vi "Read_Data_file.vi"(0 "Results file":path, 1 "Read Channel Names only":bool, 3 "Add Extra Channels?":bool, 5 "Template File":path, 8 "Desired File Types":T1) -> (10 "Row numbers":i32[](array[numeric]), 11 "Template File Out":path, 12 "Filetype":string, 13 "EOF?":bool, 14 "Results file Out":path, 15 "String Before":string, 16 "Ch names Out":string[](array[string]), 17 "Channel Values Out":string[][](array[string]), 18 "String After":string, 19 "mark after read (chars.)":i32)   [LabVIEW 2015]
uses:
  Data_File_Type.ctl
  Results_plotter_Global.vi
  Globals/Meas_global.vi
panel:
  out "Case":string
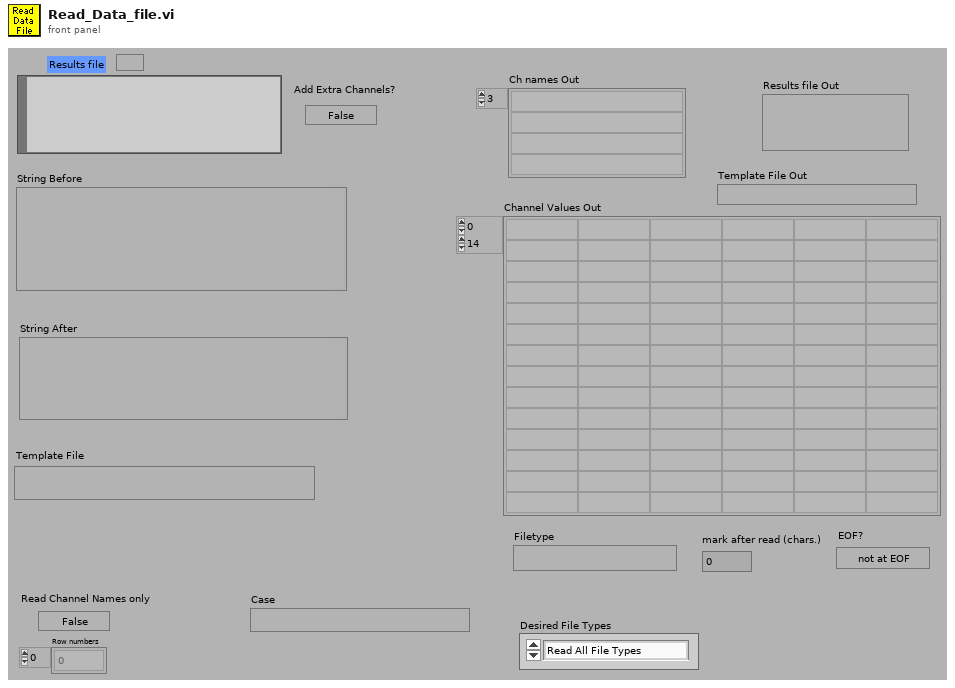
[diagram p1: front panel]
types:
  T1 = typedef "Data_File_Type.ctl" = enum16{"Read All File Types", "Results Files Only", "Raw Data Files Only", "Calibration Files Only", "Gas Desk Files Only", "Old Results Files Only", "Tabulated Data Files Only"}
  T2 = enum32{"existing file", "new file", "new or existing file", "existing dir", "new dir", "new or existing dir", "existing file (use LLBs)", "new file (use LLBs)", "new or existing file (use LLBs)", "new or existing file or directory (use LLBs)"}
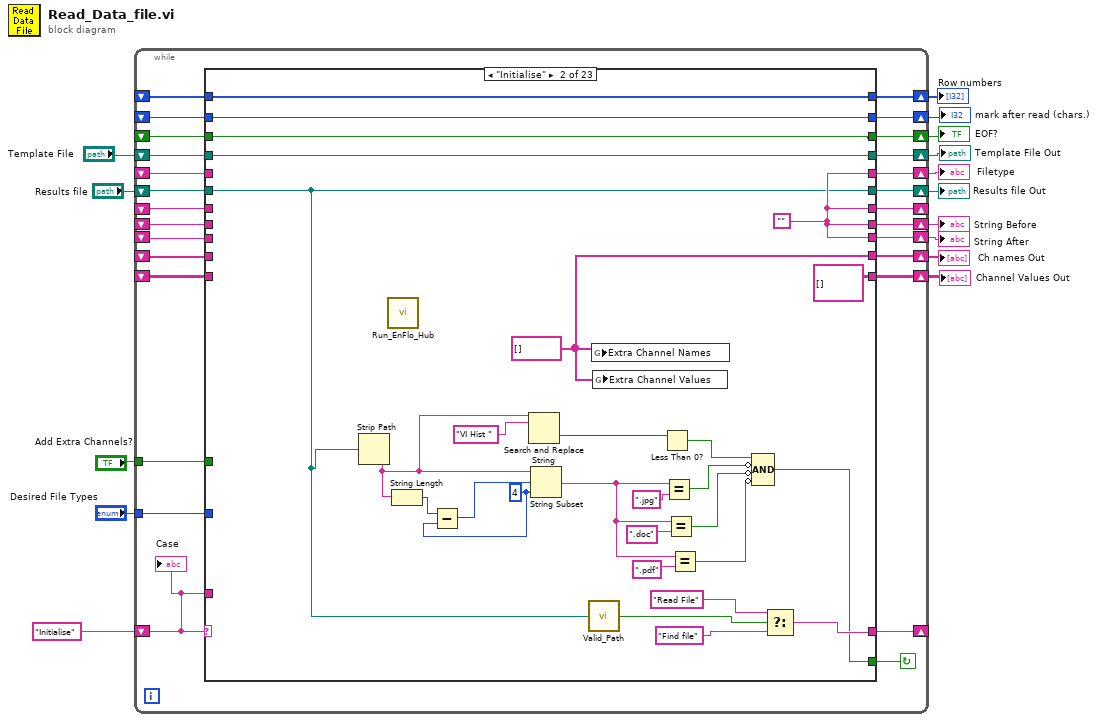
[diagram p0: block diagram]
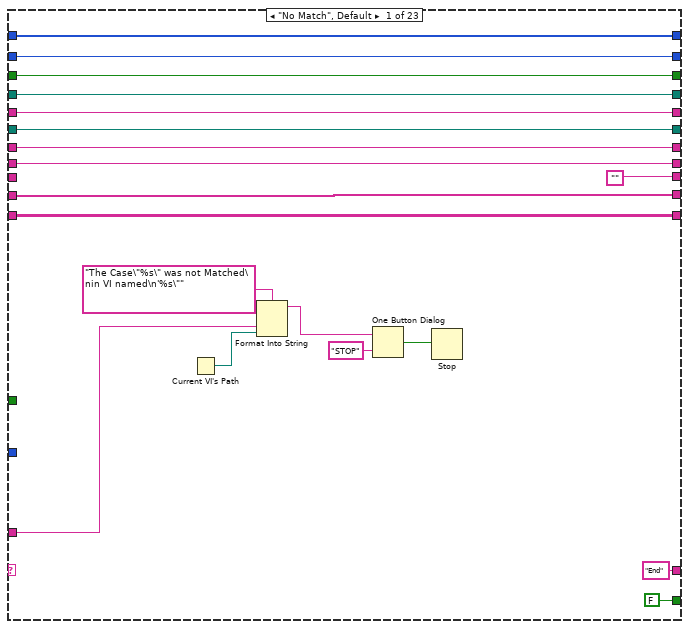
[diagram p2: hidden frame]
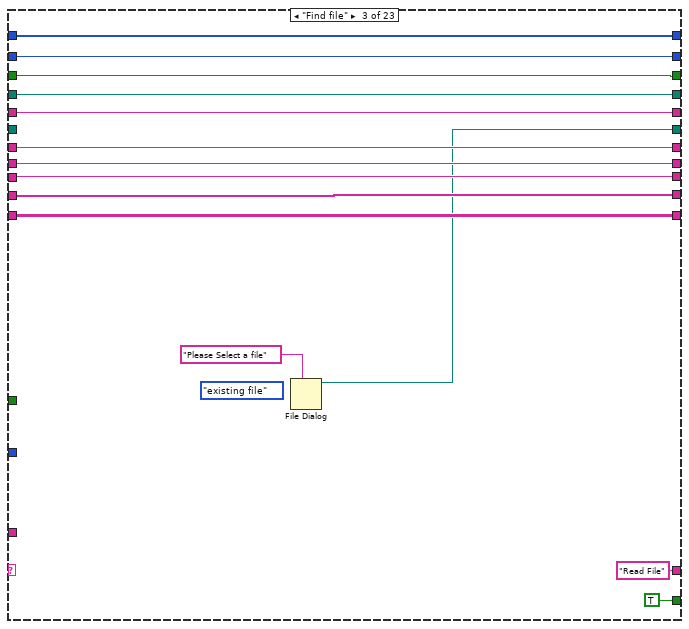
[diagram p3: hidden frame]
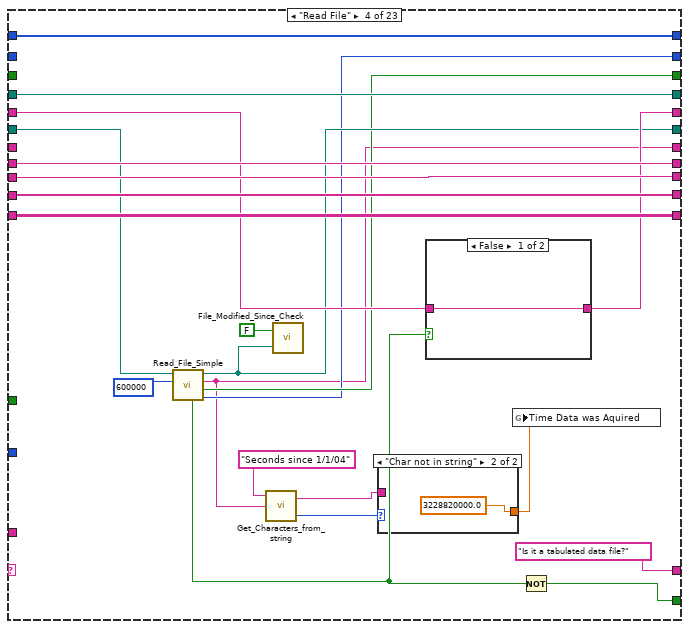
[diagram p4: hidden frame]
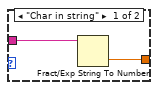
[diagram p5: hidden frame]
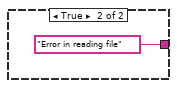
[diagram p6: hidden frame]
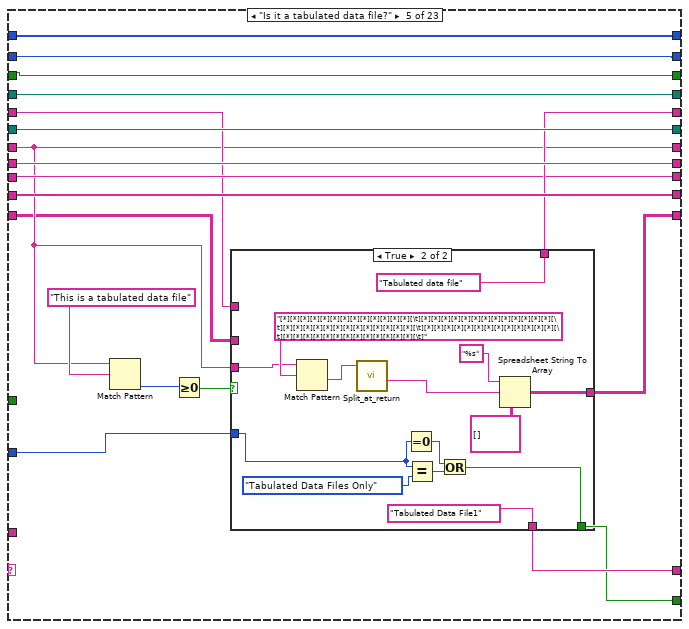
[diagram p7: hidden frame]
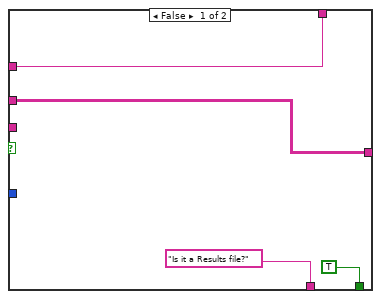
[diagram p8: hidden frame]
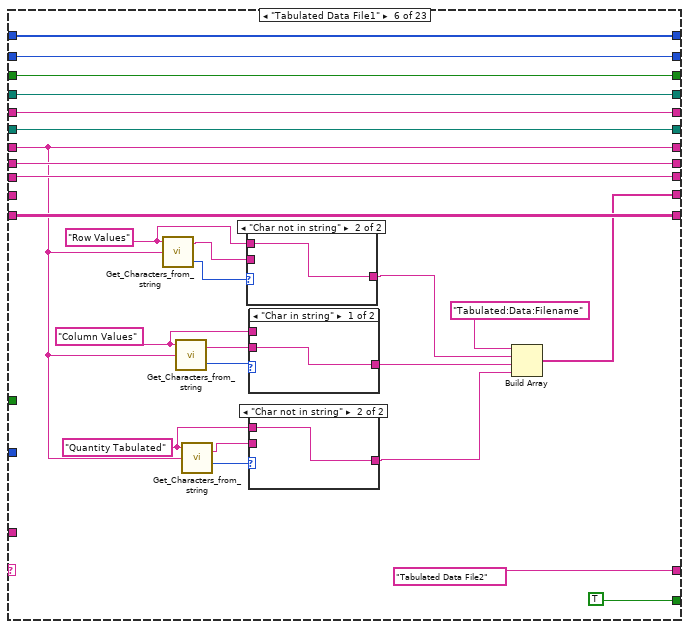
[diagram p9: hidden frame]
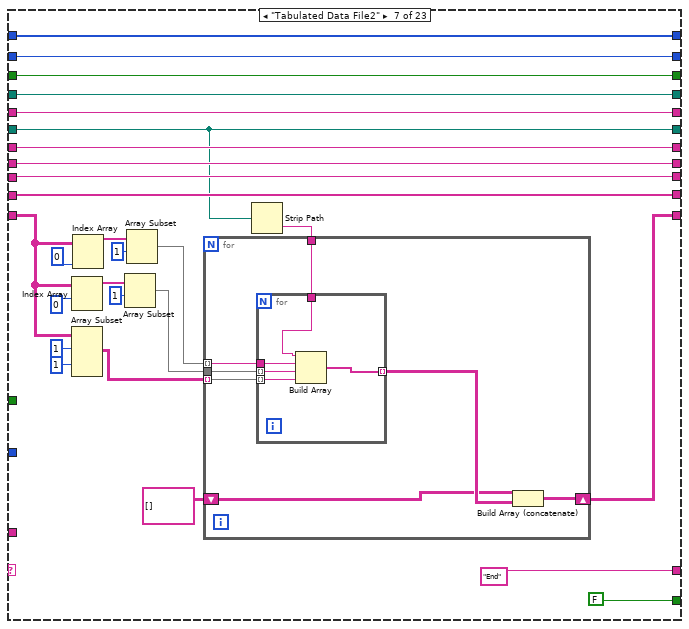
[diagram p13: hidden frame]
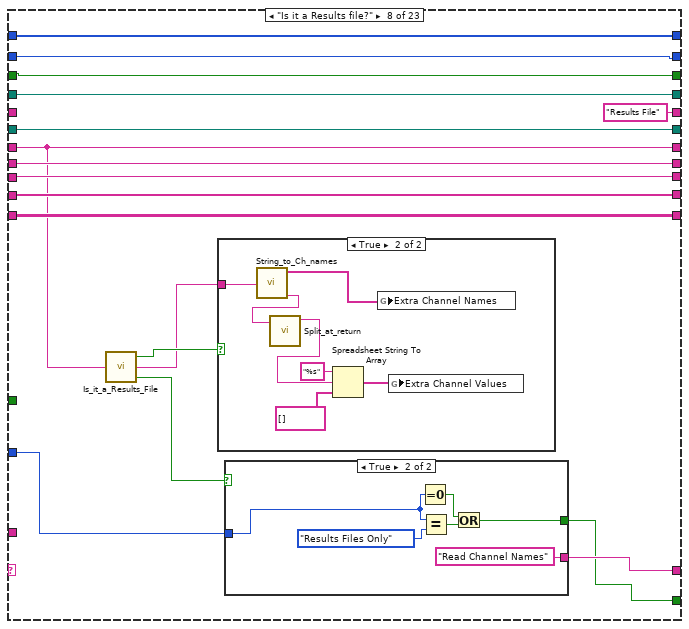
[diagram p14: hidden frame]
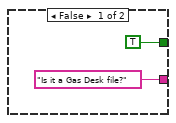
[diagram p15: hidden frame]
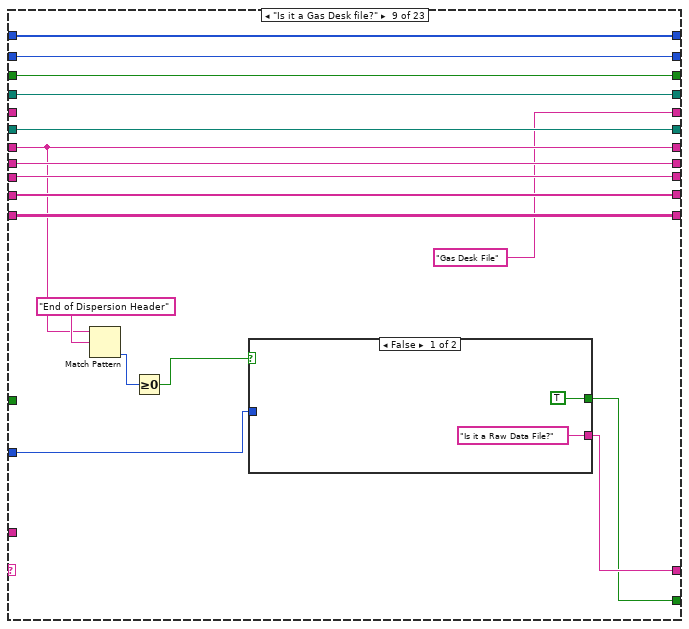
[diagram p17: hidden frame]
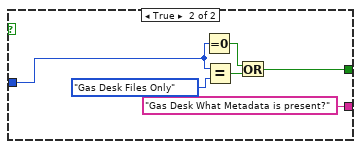
[diagram p18: hidden frame]
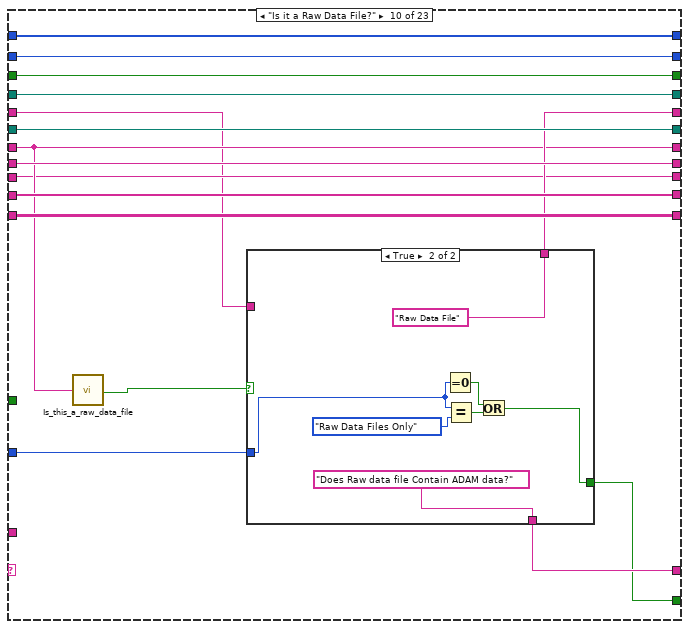
[diagram p19: hidden frame]
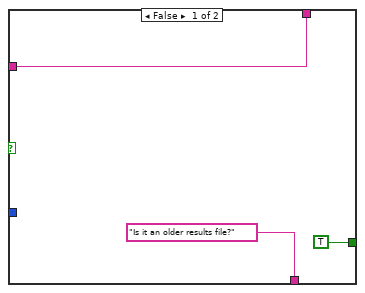
[diagram p20: hidden frame]
diagram:
  n1 = while {
    tunnel: "Add Extra Channels?" -> [w25]
    shift-left: _ -> [w29]
    shift-right: [w28] -> w14
    shift-left: "Results file" -> [w31]
    shift-right: [w30] -> w12
    shift-left: _ -> [w33]
    shift-right: [w32] -> w7
    shift-left: _ -> [w26]
    shift-right: [w34] -> w9
    shift-left: _ -> [w35]
    shift-right: [w36] -> _
    shift-left: "Initialise" -> [w39]
    shift-right: [w37] -> _
    shift-left: _ -> [w27]
    shift-right: [w41] -> w10
    shift-left: _ -> [w38]
    shift-right: [w42] -> w11
    shift-right: [w24] -> w6
    shift-left: "Template File" -> [w23]
    shift-right: [w21] -> w4
    shift-left: _ -> [w22]
    shift-right: [w20] -> w3
    shift-left: _ -> [w19]
    shift-right: [w17] -> w2
    shift-left: _ -> [w18]
    tunnel: "Desired File Types" -> [w16]
    stop <- w40 continue-if-true
    n2 = case shown="\"Initialise\"" w39 {
      tunnel: [w54 w87 w101 w123 w148 w174 w225 w254 w286 w310 w338 w372 w406 w427 w466 w494 w507 w569 w592 w628 w654 w686 w705] -> w42
      tunnel: [w53 string[][] [] ("Channel Values") w100 w122 w137 w192 w214 w253 w285 w309 w337 w371 w405 w426 w465 w493 w515 w575 w617 w627 w649 w676 w701] -> w41
      tunnel: [FALSE ("Results File?") w76 TRUE ("Results File?") w119 w130 TRUE ("Results File?") FALSE ("Results File?") w245 w270 w296 w322 w358 w398 TRUE ("Results File?") TRUE ("Results File?") TRUE ("Results File?") w501 TRUE ("Results File?") TRUE ("Results File?") FALSE ("Results File?") TRUE ("Results File?") w680 FALSE ("Results File?")] -> w40
      tunnel: w39 -> [w56 _ _ _ _ _ _ _ _ _ _ _ _ _ _ _ _ _ _ _ _ _ _]
      tunnel: w38 -> [w54 _ w101 w123 w148 _ w225 w254 w286 w310 w338 w372 w406 w427 w466 w494 _ w569 w593 w632 w654 w686 w708]
      tunnel: ["End" w88 "Read File" "Is it a tabulated data file?" w144 "Tabulated Data File2" ("f") "End" ("f") w252 w271 w305 w333 "Read Channel Names" ("f") "Read Channel Names" ("f") w412 "Read Channel Names" ("f") "Read Channel Names" ("f") w505 "Does template file exist?" ("f") w612 "End" ("f") "Delete First Row?" ("f") "Add Extra Channels of data" ("f") "End" ("f")] -> w37
      tunnel: [w51 w85 w98 w105 w138 w185 w221 w247 w279 w303 w328 w367 w394 w414 w444 w477 w508 w570 w616 w633 w647 w688 w710] -> w36
      tunnel: w35 -> [w51 _ w98 _ w138 w185 w221 w247 w279 w303 w328 w367 w401 w413 w444 w477 w510 w570 w616 w633 w647 w688 w710]
      tunnel: [w50 w85 w97 w121 w146 w190 w224 w248 w282 w307 w335 w370 w403 w423 w462 w491 w509 w567 w615 w636 w653 w691 w714] -> w34
      tunnel: w33 -> [_ _ w96 w120 w143 w188 w222 w250 w283 w302 w332 w369 _ w424 w463 w492 w514 w574 w614 w635 w652 w690 w713]
      tunnel: ["" w85 w96 w120 w143 w188 w222 w250 w283 w302 w332 w369 w391 w424 w463 w492 w514 w574 w614 w635 w652 w690 w713] -> w32
      tunnel: w31 -> [w49 w69 _ w116 w147 w191 w204 w251 w284 w308 w336 w350 w404 w425 w464 w471 w513 w573 w610 w631 w646 w687 w709]
      tunnel: [w49 w69 w95 w112 w147 w191 w204 w251 w284 w308 w336 w350 w404 w425 w464 w471 w513 w573 w610 w631 w646 w687 w709] -> w30
      tunnel: w29 -> [w47 _ w93 w117 w142 w187 w220 _ _ w301 w331 _ w397 w411 w460 w489 w512 w572 w613 w630 w643 w685 w712]
      tunnel: [w47 w85 w93 w118 w145 w187 w220 "Results File" "Gas Desk File" w306 w334 w357 w397 w411 w460 w489 w512 w572 w613 w630 w643 w685 w712] -> w28
      tunnel: w27 -> [w53 _ w100 w122 w136 w192 w213 w253 w285 w309 w337 w371 w405 w426 w465 w493 w515 w575 w617 _ _ w684 w703]
      tunnel: w26 -> [w50 _ w97 w121 w146 w190 w224 w248 w282 w307 w335 w370 w403 w423 w462 w491 _ w567 w615 w636 w653 w691 w714]
      tunnel: w25 -> [_ _ _ _ _ _ _ _ _ _ _ w359 _ _ _ _ _ _ _ _ _ w671 _]
      tunnel: [w46 w75 w92 w111 w135 w170 w202 w243 w277 w300 w326 w356 w388 w410 w442 w470 w503 w565 w595 w626 w642 w679 w700] -> w24
      tunnel: w23 -> [w46 w75 w92 w111 w135 w170 w202 w243 w277 w300 w326 w356 w388 w410 w442 w470 w503 w565 w595 w625 w642 w679 w700]
      tunnel: w22 -> [w44 w73 w90 _ w133 w168 w200 w241 w275 w298 w324 w354 w386 w408 w440 w468 w502 w564 w604 w624 w641 w677 w698]
      tunnel: [w44 w73 w90 w110 w133 w168 w200 w241 w275 w298 w324 w354 w386 w408 w440 w468 w502 w564 w604 w624 w640 w677 w698] -> w21
      tunnel: [w45 w74 w91 w109 w134 w169 w201 w242 w276 w299 w325 w355 w387 w409 w441 w469 w498 w563 w603 w623 w639 w678 w699] -> w20
      tunnel: w19 -> [w45 w74 w91 _ w134 w169 w201 w242 w276 w299 w325 w355 w387 w409 w441 w469 w499 w563 w603 w623 w639 w678 w699]
      tunnel: [w43 w72 w89 w108 w132 w167 w199 w240 w274 w297 w323 w353 w385 w407 w439 w467 w495 w562 w602 w622 w638 w672 w697] -> w17
      tunnel: w18 -> [w43 w72 w89 w108 w132 w167 w199 w240 w274 w297 w323 w353 w385 w407 w439 w467 w495 w562 w602 _ w638 _ w697]
      tunnel: w16 -> [_ _ _ _ w131 _ _ w238 w273 w295 w321 w352 _ _ _ _ _ _ _ _ _ _ _]
      frame "No Match", Default {
        n3 = Current VI's Path() -> (path=w57:path)
        n4 = Format Into String(format string="The Case\"%s\" was not Matched\nin VI named\n'%s\"" ("Format String"), w56, w57) -> (resulting string=w60:string)  [unwired: 2 in, 1 out]
        n5 = One Button Dialog(message=w60, button name ("OK")="STOP") -> (true=w58:bool)
        n6 = Stop(stop? (T)=w58) -> ()
      }
      frame "Initialise" {
        w83 = 4 ("length (rest)")
        w85 = ""
        w87 = string[] [] ("Extra Channel Names")
        n7 = Strip Path(path=w69) -> (name=w81:string)  [unwired: 1 out]
        n8 = call "Run_EnFlo_Hub.vi"() -> ()  [unwired: 1 in, 7 out]
        n9 = String Length(string=w81) -> (length=w84:i32)
        n10 = Subtract(x=w84, y=w83) -> (x-y=w82:i32)
        n11 = Search and Replace String(input string=w81, search string="VI Hist ") -> (offset past replacement=w79:i32)  [unwired: 1 in, 8 out]
        n12 = String Subset(string=w81, offset (0)=w82, length (rest)=w83) -> (substring=w63:string)
        n13 = call "Valid_Path.vi"("Filename"=w69) -> ("Valid Path?"=w68:bool)
        n14 = global write "Results_plotter_Global.vi" "Extra Channel Names"(w87) -> ()
        n15 = global write "Results_plotter_Global.vi" "Extra Channel Values"(w87) -> ()
        n16 = Less Than 0?(x=w79) -> (x < 0?=w77:bool)
        n17 = Equal?(x=w63, y=".jpg") -> (x = y?=w78:bool)
        n18 = Equal?(x=w63, y=".doc") -> (x = y?=w66:bool)
        n19 = Equal?(x=w63, y=".pdf") -> (x = y?=w62:bool)
        n20 = Compound Arithmetic op=AND(w77, invert w78, invert w66, invert w62) -> (w76:bool)
        n21 = Select(t="Read File", s=w68, f="Find file") -> (s? t:f=w88:string)
      }
      frame "Find file" {
        (unwired) T2."existing file" ("select mode (2)")
        n22 = File Dialog(7:"Please Select a file" ("prompt")) -> (3:w95:path)  [unwired: 1 in, 8 out]
      }
      frame "Read File" {
        n23 = call "Read_File_Simple.vi"("Filename"=w116, "number of characters (all:-1)"=600000 ("count")) -> ("Error?"=w114:bool, "Filename Out"=w112:path, "string"=w105:string, "EOF?"=w110:bool, "mark after read (chars.)"=w109:i32)  [unwired: 1 in, 3 out]
        n24 = call "Get_Characters_from_string.vi"("Input string"=w105, "Variable name"="Seconds since 1/1/04") -> ("Status"=w103:enum16{"Char in string", "Char not in string"}, "Value"=w106:string)  [unwired: 1 in]
        n25 = call "File_Modified_Since_Check.vi"("Pathname"=w112, "Just Modified?"=FALSE) -> ()  [unwired: 1 out]
        n26 = case shown="\"Char not in string\"" w103 {
          tunnel: w106 -> [w126 _]
          tunnel: [w125 3228820000.0 ("y")] -> w104
          frame "Char in string" {
            n27 = Fract/Exp String To Number(string=w126) -> (number=w125:dbl)  [unwired: 4 out]
          }
          frame "Char not in string" {
          }
        }
        n28 = case shown="False" w114 {
          tunnel: [w128 "Error in reading file"] -> w118
          tunnel: w117 -> [w128 _]
          frame False {
          }
          frame True {
          }
        }
        n29 = global write "Meas_global.vi" "Time Data was Aquired"(w104) -> ()
        n30 = Not(x=w114) -> (.not. x?=w119:bool)
      }
      frame "Is it a tabulated data file?" {
        n31 = Match Pattern(string=w138, regular expression="This is a tabulated data file") -> (offset past match=w141:i32)  [unwired: 4 out]
        n32 = Greater Or Equal To 0?(x=w141) -> (x >= 0?=w140:bool)
        n33 = case shown="True" w140 {
          tunnel: [w152 "Tabulated data file"] -> w145
          tunnel: ["Is it a Results file?" "Tabulated Data File1" ("f")] -> w144
          tunnel: w142 -> [w152 _]
          tunnel: w138 -> [_ w163]
          tunnel: [w151 w160] -> w137
          tunnel: w136 -> [w151 _]
          tunnel: w131 -> [_ w156]
          tunnel: [TRUE ("Results File?") w153] -> w130
          frame False {
          }
          frame True {
            n34 = Match Pattern(string=w163, regular expression="[*][*][*][*][*][*][*][*][*][*][*][*][*][\t][*][*][*][*][*][*][*][*][*][*][*][*][*][\t][*][*][*][*][*][*][*][*][*][*][*][*][*][\t][*][*][*][*][*][*][*][*][*][*][*][*][*][\t][*][*][*][*][*][*][*][*][*][*][*][*][*][\t]" ("String")) -> (after substring=w159:string)  [unwired: 4 out]
            n35 = call "Split_at_return.vi"("String"=w159) -> ("after substring"=w158:string)  [unwired: 1 in, 3 out]
            n36 = Equal To 0?(x=w156) -> (x = 0?=w154:bool)
            n37 = Equal?(x=w156, y=Data_File_Type."Tabulated Data Files Only" ("Desired File Types")) -> (x = y?=w155:bool)
            n38 = Or(x=w154, y=w155) -> (x .or. y?=w153:bool)
            n39 = Spreadsheet String To Array(format string="%s", spreadsheet string=w158, array type (2D Dbl)=string[][] [] ("Channel Values")) -> (array=w160:string[][])  [unwired: 1 out]
          }
        }
      }
      frame "Tabulated Data File1" {
        w173 = "Row Values" ("Variable name")
        w172 = "Column Values" ("Variable name")
        w179 = "Quantity Tabulated" ("Variable name")
        n40 = call "Get_Characters_from_string.vi"("Input string"=w185, "Variable name"=w173) -> ("Status"=w177:enum16{"Char in string", "Char not in string"}, "Value"=w178:string)  [unwired: 1 in]
        n41 = call "Get_Characters_from_string.vi"("Input string"=w185, "Variable name"=w172) -> ("Status"=w184:enum16{"Char in string", "Char not in string"}, "Value"=w183:string)  [unwired: 1 in]
        n42 = call "Get_Characters_from_string.vi"("Input string"=w185, "Variable name"=w179) -> ("Status"=w181:enum16{"Char in string", "Char not in string"}, "Value"=w180:string)  [unwired: 1 in]
        n43 = case shown="\"Char not in string\"" w177 {
          tunnel: w178 -> [w195 _]
          tunnel: [w195 w196] -> w176
          tunnel: w173 -> [_ w196]
          frame "Char in string" {
          }
          frame "Char not in string" {
          }
        }
        n44 = case shown="\"Char in string\"" w184 {
          tunnel: w183 -> [w197 _]
          tunnel: [w197 w198] -> w182
          tunnel: w172 -> [_ w198]
          frame "Char in string" {
          }
          frame "Char not in string" {
          }
        }
        n45 = case shown="\"Char not in string\"" w181 {
          tunnel: w180 -> [w193 _]
          tunnel: [w193 w194] -> w175
          tunnel: w179 -> [_ w194]
          frame "Char in string" {
          }
          frame "Char not in string" {
          }
        }
        n46 = Build Array("Tabulated:Data:Filename", w176, w182, w175) -> (w174:string[])
      }
      frame "Tabulated Data File2" {
        n47 = Index Array(array=w213, index (row)=0) -> (element=w212:string[])  [unwired: 1 in]
        n48 = Array Subset(array=w213, index (row)=1 ("index"), index (col)=1 ("index")) -> (w216:string[][])  [unwired: 2 in]
        n49 = Index Array(array=w213, index (col)=0 ("index (row)")) -> (element=w208:string[])  [unwired: 1 in]
        n50 = Array Subset(array=w212, index=1) -> (w209:string[])  [unwired: 1 in]
        n51 = Array Subset(array=w208, index=1) -> (w207:string[])  [unwired: 1 in]
        n52 = Strip Path(path=w204) -> (name=w203:string)  [unwired: 1 out]
        n53 = for {
          tunnel: w207 -> [w232] mode=indexing
          tunnel: w209 -> [w231]
          tunnel: w216 -> [w230] mode=indexing
          shift-right: [w227] -> w214
          shift-left: string[][] [] -> [w228]
          tunnel: w203 -> [w226]
          n54 = for {
            tunnel: w232 -> [w237]
            tunnel: w231 -> [w236] mode=indexing
            tunnel: w230 -> [w235] mode=indexing
            tunnel: [w234] -> w229 mode=indexing
            tunnel: w226 -> [w233]
            n55 = Build Array(w233, w237, w236, w235) -> (w234:string[])
          }
          n56 = Build Array (concatenate)(w228, w229) -> (w227:string[][])
        }
      }
      frame "Is it a Results file?" {
        n57 = call "Is_it_a_Results_File.vi"("character string"=w247) -> ("Contain DB Header Info"=w246:bool, "Header String"=w239:string, "Results File?"=w244:bool)
        n58 = case shown="True" w246 {
          tunnel: w239 -> [_ w265]
          frame False {
          }
          frame True {
            n59 = call "String_to_Ch_names.vi"("Spreadsheet string"=w265) -> ("Ch names"=w264:string[], "String After names"=w268:string)  [unwired: 2 out]
            n60 = call "Split_at_return.vi"("String"=w268) -> ("before substring"=w269:string)  [unwired: 1 in, 3 out]
            n61 = Spreadsheet String To Array(format string="%s", spreadsheet string=w269, array type (2D Dbl)=string[] [] ("Channel Values")) -> (array=w263:string[])  [unwired: 1 out]
            n62 = global write "Results_plotter_Global.vi" "Extra Channel Names"(w264) -> ()
            n63 = global write "Results_plotter_Global.vi" "Extra Channel Values"(w263) -> ()
          }
        }
        n64 = case shown="True" w244 {
          tunnel: ["Is it a Gas Desk file?" "Read Channel Names"] -> w252
          tunnel: w238 -> [_ w259]
          tunnel: [TRUE w257] -> w245
          frame False {
          }
          frame True {
            n65 = Equal To 0?(x=w259) -> (x = 0?=w260:bool)
            n66 = Equal?(x=w259, y=Data_File_Type."Results Files Only" ("Desired File Types")) -> (x = y?=w261:bool)
            n67 = Or(x=w260, y=w261) -> (x .or. y?=w257:bool)
          }
        }
      }
      frame "Is it a Gas Desk file?" {
        n68 = Match Pattern(string=w279, regular expression="End of Dispersion Header") -> (offset past match=w281:i32)  [unwired: 4 out]
        n69 = Greater Or Equal To 0?(x=w281) -> (x >= 0?=w272:bool)
        n70 = case shown="False" w272 {
          tunnel: ["Is it a Raw Data File?" "Gas Desk What Metadata is present?"] -> w271
          tunnel: w273 -> [_ w291]
          tunnel: [TRUE w289] -> w270
          frame False {
          }
          frame True {
            n71 = Equal To 0?(x=w291) -> (x = 0?=w292:bool)
            n72 = Equal?(x=w291, y=Data_File_Type."Gas Desk Files Only" ("Desired File Types")) -> (x = y?=w293:bool)
            n73 = Or(x=w292, y=w293) -> (x .or. y?=w289:bool)
          }
        }
      }
      frame "Is it a Raw Data File?" {
        n74 = call "Is_this_a_raw_data_file.vi"("character string"=w303) -> ("Raw Dat File?"=w304:bool)  [unwired: 2 out]
        n75 = case shown="True" w304 {
          tunnel: [w312 "Raw Data File"] -> w306
          tunnel: ["Is it an older results file?" ("f") "Does Raw data file Contain ADAM data?" ("f")] -> w305
          tunnel: w301 -> [w312 _]
          tunnel: [TRUE ("Results File?") w315] -> w296
          tunnel: w295 -> [_ w316]
          frame False {
          }
          frame True {
            n76 = Equal To 0?(x=w316) -> (x = 0?=w318:bool)
            n77 = Equal?(x=w316, y=Data_File_Type."Raw Data Files Only" ("Desired File Types")) -> (x = y?=w317:bool)
            n78 = Or(x=w318, y=w317) -> (x .or. y?=w315:bool)
          }
        }
      }
      frame "Is it an older results file?" {
        n79 = Match Pattern(string=w328, regular expression="Date of meas\tTime of meas") -> (offset past match=w329:i32)  [unwired: 4 out]
        n80 = Greater Or Equal To 0?(x=w329) -> (x >= 0?=w327:bool)
        n81 = case shown="True" w327 {
          tunnel: [w341 "Older Results File"] -> w334
          tunnel: ["Is it a calibration file?" ("f") "Read Channel Names" ("f")] -> w333
          tunnel: w331 -> [w341 _]
          tunnel: [TRUE ("Results File?") w343] -> w322
          tunnel: w321 -> [_ w342]
          frame False {
          }
          frame True {
            n82 = Equal To 0?(x=w342) -> (x = 0?=w346:bool)
            n83 = Equal?(x=w342, y=Data_File_Type."Old Results Files Only" ("Desired File Types")) -> (x = y?=w345:bool)
            n84 = Or(x=w346, y=w345) -> (x .or. y?=w343:bool)
          }
        }
      }
      frame "Is it a calibration file?" {
        w366 = FALSE  # Show Dialog?
        n85 = Format Into String(format string="Data File   %s", w350) -> (resulting string=w349:string)  [unwired: 2 in, 1 out]
        n86 = call "2D_array_from_string.vi"("String Name"=w349, "Show Dialog?"=w366, "Input string"=w367, "Array title"="Calib points label") -> ("2D data array"=w365:dbl[][])
        n87 = Array Size(array=w365) -> (size(s)=w364:i32[])
        n88 = Index Array(array=w364, index=0 ("Index")) -> (element=w362:i32)
        n89 = Greater Than 0?(x=w362) -> (x > 0?=w360:bool)
        n90 = case shown="False" w360 {
          tunnel: w359 -> [_ w384]
          tunnel: [w373 w376] -> w358
          tunnel: ["File with no header" "Calibration File"] -> w357
          tunnel: w352 -> [w374 w380]
          frame False {
            n91 = Equal To 0?(x=w374) -> (x = 0?=w373:bool)
          }
          frame True {
            n92 = Not(x=w384) -> (.not. x?=w377:bool)
            n93 = Equal To 0?(x=w380) -> (x = 0?=w382:bool)
            n94 = Equal?(x=w380, y=Data_File_Type."Calibration Files Only" ("Desired File Types")) -> (x = y?=w381:bool)
            n95 = Or(x=w382, y=w381) -> (x .or. y?=w378:bool)
            n96 = Or(x=w378, y=w377) -> (x .or. y?=w376:bool)
          }
        }
      }
      frame "Does Raw data file Contain ADAM data?" {
        w389 = "\r\n"
        w392 = "Raw data header Start"
        n97 = Match Pattern(string=w401, regular expression=w392) -> (before substring=w395:string, after substring=w390:string)  [unwired: 3 out]
        n98 = Match Pattern(string=w395, regular expression="[*][*][*][*][*][*][*][*][*][*][*][*][*][*][*][*][*][*][*][*][*]" ("String")) -> (before substring=w394:string)  [unwired: 4 out]
        n99 = Concatenate Strings(w389, "************************", w389, w392, w390) -> (w391:string)
        n100 = String Length(string=w395) -> (length=w400:i32)
        n101 = Greater?(x=w400, y=30) -> (0:w398:bool)
      }
      frame "Gas Desk What Metadata is present?" {
        n102 = String Subset(string=w413, offset (0)=0, length (rest)=6 ("length")) -> (substring=w420:string)
        n103 = Equal?(x="******", y=w420) -> (x = y?=w418:bool)
        n104 = case shown="False" w418 {
          tunnel: [w429 "Gas Desk Read ADAM ch's Header"] -> w412
          tunnel: w413 -> [w428 _]
          frame False {
            w433 = "Data Base\tData Base\tData Base\t"
            n105 = String Length(string=w433) -> (length=w436:i32)
            n106 = String Subset(string=w428, offset (0)=0, length (rest)=w436) -> (substring=w434:string)
            n107 = Equal?(x=w433, y=w434) -> (x = y?=w432:bool)
            n108 = Select(t="Gas Desk DB Header Present", s=w432, f="Read Channel Names") -> (s? t:f=w429:string)
          }
          frame True {
          }
        }
        n109 = call "Fast_string_Replace.vi"("Replace match with:"="Suspect Pulse Width" ("regular expression"), "Input String"=w413, "regular expression"="Suspect \u0003Pulse Width ") -> ("Output String"=w414:string)  [unwired: 2 out]
      }
      frame "Gas Desk DB Header Present" {
        w447 = string[] [] ("Channel Values")
        n110 = call "String_to_Ch_names.vi"("Spreadsheet string"=w444) -> ("Ch names"=w459:string[], "String After names"=w448:string)  [unwired: 2 out]
        n111 = call "Split_at_return.vi"("String"=w448) -> ("before substring"=w450:string, "after substring"=w451:string)  [unwired: 1 in, 2 out]
        n112 = call "Split_at_return.vi"("String"=w451) -> ("after substring"=w452:string)  [unwired: 1 in, 3 out]
        n113 = call "String_to_Ch_names.vi"("Spreadsheet string"=w452) -> ("Ch names"=w458:string[], "String After names"=w453:string)  [unwired: 2 out]
        n114 = call "Split_at_return.vi"("String"=w453) -> ("after substring"=w455:string)  [unwired: 1 in, 3 out]
        n115 = call "Split_at_return.vi"("String"=w455) -> ("before substring"=w456:string)  [unwired: 1 in, 3 out]
        n116 = Spreadsheet String To Array(format string="%s", spreadsheet string=w450, array type (2D Dbl)=w447) -> (array=w446:string[])  [unwired: 1 out]
        n117 = Spreadsheet String To Array(format string="%s", spreadsheet string=w456, array type (2D Dbl)=w447) -> (array=w457:string[])  [unwired: 1 out]
        n118 = Build Array (concatenate)(w458, w459) -> (w438:string[])
        n119 = Build Array (concatenate)(w457, w446) -> (w445:string[])
        n120 = global write "Results_plotter_Global.vi" "Extra Channel Values"(w445) -> ()
        n121 = global write "Results_plotter_Global.vi" "Extra Channel Names"(w438) -> ()
      }
      frame "Gas Desk Read ADAM ch's Header" {
        n122 = call "Split_at_return.vi"("String"=w477) -> ("after substring"=w485:string)  [unwired: 1 in, 3 out]
        n123 = call "String_to_Ch_names.vi"("Spreadsheet string"=w485) -> ("Ch names"=w473:string[], "String After names"=w486:string)  [unwired: 2 out]
        n124 = call "Split_at_return.vi"("String"=w486) -> ("after substring"=w487:string)  [unwired: 1 in, 3 out]
        n125 = call "Split_at_return.vi"("String"=w487) -> ("before substring"=w484:string)  [unwired: 1 in, 3 out]
        n126 = Spreadsheet String To Array(format string="%s", spreadsheet string=w484, array type (2D Dbl)=string[] [] ("Channel Values")) -> (array=w478:string[])  [unwired: 1 out]
        n127 = Strip Path(path=w471) -> (stripped path=w480:path, name=w479:string)
        n128 = Path To String(path=w480) -> (string=w481:string)
        n129 = Build Array (concatenate)("Original:Results:Filename", "Original:Results:Filepath", w473) -> (w472:string[])
        n130 = Build Array (concatenate)(w479, w481, w478) -> (w476:string[])
        n131 = global write "Results_plotter_Global.vi" "Extra Channel Names"(w472) -> ()
        n132 = global write "Results_plotter_Global.vi" "Extra Channel Values"(w476) -> ()
      }
      frame "Read Channel Names" {
        n133 = case shown="\"Older Results File\"" w512 {
          tunnel: [w523 w537 w546 0 0] -> w496
          tunnel: [w522 w536 w550 w555 w560] -> w506
          tunnel: w510 -> [w521 w538 w549 w558 w560]
          tunnel: [w520 w544 "Is Raw Data Filename Present?" ("f") w553 w559] -> w505
          tunnel: "Does template file exist?" ("f") -> [w520 w544 _ w553 w559]
          frame "Results File" {
            n134 = Match Pattern(string=w521, regular expression="[*][*][*][*][*][*][*][*][*][*][*][*][*][\t][*][*][*][*][*][*][*][*][*][*][*][*][*][\t][*][*][*][*][*][*][*][*][*][*][*][*][*][\t][*][*][*][*][*][*][*][*][*][*][*][*][*][\t][*][*][*][*][*][*][*][*][*][*][*][*][*][\t]" ("String")) -> (after substring=w526:string, offset past match=w524:i32)  [unwired: 3 out]
            n135 = call "Split_at_return.vi"("String"=w526) -> ("after substring"=w522:string, "offset past match"=w525:i32)  [unwired: 1 in, 2 out]
            n136 = Add(x=w524, y=w525) -> (x+y=w523:i32)
          }
          frame "Older Results File" {
            w531 = "\r"
            n137 = Match Pattern(string=w538, regular expression="Date of meas\tTime of meas") -> (before substring=w542:string, match substring=w535:string, offset past match=w539:i32)  [unwired: 2 out]
            n138 = Reverse String(1:w542) -> (0:w541:string)
            n139 = String Length(string=w535) -> (length=w534:i32)
            n140 = Match Pattern(string=w541, regular expression=w531) -> (after substring=w540:string, offset past match=w532:i32)  [unwired: 3 out]
            n141 = Match Pattern(string=w540, regular expression=w531) -> (after substring=w530:string, offset past match=w533:i32)  [unwired: 3 out]
            n142 = Match Pattern(string=w530, regular expression=w531) -> (offset past match=w529:i32)  [unwired: 4 out]
            n143 = Compound Arithmetic op=ADD(invert w534, w539, invert w533, invert w532, invert w529, 1 ("value")) -> (w537:i32)
            n144 = Search/Split String(string=w538, offset (0)=w537) -> (match + rest of string=w536:string)  [unwired: 3 out]
          }
          frame "Gas Desk File" {
            n145 = Match Pattern(string=w549, regular expression="End of Dispersion Header") -> (after substring=w552:string, offset past match=w547:i32)  [unwired: 3 out]
            n146 = call "Split_at_return.vi"("String"=w552) -> ("after substring"=w550:string, "offset past match"=w548:i32)  [unwired: 1 in, 2 out]
            n147 = Add(x=w548, y=w547) -> (x+y=w546:i32)
          }
          frame "Raw Data File" {
            n148 = Search/Split String(string=w558, offset (0)=37 ("y")) -> (match + rest of string=w557:string)  [unwired: 3 out]
            n149 = call "Split_at_return.vi"("String"=w557) -> ("after substring"=w555:string)  [unwired: 1 in, 3 out]
          }
          frame "File with no header", Default {
          }
        }
        n150 = call "String_to_Ch_names.vi"("Spreadsheet string"=w506) -> ("Ch names"=w507:string[], "Title length (Bytes)"=w497:i32, "String After names"=w508:string)  [unwired: 1 out]
        n151 = case shown="True" "Read Channel Names only" {
          tunnel: w499 -> [w516 _]
          tunnel: [w516 w517] -> w498
          tunnel: w497 -> [_ w519]
          tunnel: w496 -> [_ w518]
          frame False {
          }
          frame True {
            n152 = Add(x=w518, y=w519) -> (x+y=w517:i32)
          }
        }
        n153 = String Subset(string=w510, offset (0)=0, length (rest)=w496) -> (substring=w509:string)
        n154 = Not(x="Read Channel Names only") -> (.not. x?=w501:bool)
      }
      frame "Is Raw Data Filename Present?" {
        w566 = "Raw:Data:Filename"
        n155 = Search 1D Array(1D array=w569, element=w566) -> (index of element=w568:i32)  [unwired: 1 out]
        n156 = case shown="-1" w568 {
          tunnel: w567 -> [_ w589]
          tunnel: w566 -> [_ w583]
          frame 0, Default {
          }
          frame -1 {
            n157 = global read "Results_plotter_Global.vi" "Extra Channel Names"() -> (w584:string[])
            n158 = global read "Results_plotter_Global.vi" "Extra Channel Values"() -> (w582:string[])
            n159 = Concatenate Strings("Raw data Directory", "\t") -> (w586:string)
            n160 = Match Pattern(string=w589, regular expression=w586) -> (after substring=w585:string)  [unwired: 4 out]
            n161 = call "Split_at_return.vi"("String"=w585) -> ("before substring"=w578:string)  [unwired: 1 in, 3 out]
            n162 = Build Array (concatenate)(w584, w583) -> (w580:string[])
            n163 = global write "Results_plotter_Global.vi" "Extra Channel Names"(w580) -> ()
            n164 = Match Pattern(string=w578, regular expression="\t") -> (before substring=w577:string)  [unwired: 4 out]
            n165 = Build Array (concatenate)(w582, w577) -> (w581:string[])
            n166 = global write "Results_plotter_Global.vi" "Extra Channel Values"(w581) -> ()
          }
        }
      }
      frame "Does template file exist?" {
        n167 = global read "Results_plotter_Global.vi" "Extra Channel Names"() -> (w611:string[])
        n168 = while {
          shift-right: [w620] -> w599
          shift-left: _ -> [w621]
          stop <- TRUE stop-if-true
          n169 = Increment(x=w621) -> (x+1=w620:dbl)
        }
        n170 = call "Common_Extra_Chs.vi"() -> ("Common Extra Channels"=w601:string[])
        n171 = call "Valid_Path.vi"("Filename"=w595) -> ("Valid Path?"=w594:bool)
        n172 = Path to Array of Strings(0:w610) -> (2:w609:string[])  [unwired: 1 out]
        n173 = global read "Results_plotter_Global.vi" "Extra Channel Values"() -> (w607:string[])
        n174 = Build Array (concatenate)(w611, w601) -> (w591:string[])
        n175 = Reverse 1D Array(array=w609) -> (reversed array=w608:string[])
        n176 = call "Update_Ch_Names.vi"("Ch Name in"=w591) -> ("Ch Name Out"=w590:string[])
        n177 = Array Subset(array=w608, length=5) -> (w606:string[])  [unwired: 1 in]
        n178 = Number To Decimal String(number=w599) -> (decimal integer string=w598:string)  [unwired: 1 out]
        n179 = Select(t="Read Values using Template", s=w594, f="Entire string to 2D array") -> (s? t:f=w612:string)
        n180 = Build Array (concatenate)(w607, w606, w598) -> (w605:string[])
        n181 = global write "Results_plotter_Global.vi" "Extra Channel Names"(w590) -> ()
        n182 = call "Update_Ch_Names.vi"("Ch Name in"=w593) -> ("Ch Name Out"=w592:string[])
        n183 = global write "Results_plotter_Global.vi" "Extra Channel Values"(w605) -> ()
      }
      frame "Read Values using Template" {
        n184 = call "Filter_on_template_file_new.vi"("Filetype"=w630, "Filename"=w631, "End Of File already Reached?"=w624, "Start of data (bytes)"=w623, "Data string"=w633, "Channel Names In"=w632, "Template File"=w625) -> ("Data Out"=w629:string[][], "Channel Names Out"=w628:string[], "Row numbers"=w622:i32[], "Template File-write"=w626:path)  [unwired: 1 out]
        n185 = call "Surface_modularity.vi"("Data in"=w629, "Channel names"=w628) -> ("Data out"=w627:string[][])  [unwired: 1 out]
      }
      frame "Entire string to 2D array" {
        n186 = case shown="\"False\", Default" w643 {
          tunnel: [w660 w670] -> w648
          tunnel: w647 -> [w659 w670]
          tunnel: w646 -> [w658 _]
          tunnel: w641 -> [w656 w669]
          tunnel: [w657 w669] -> w640
          tunnel: w639 -> [w655 _]
          frame "False", Default {
            n187 = case shown="False" w656 {
              tunnel: [w664 w668] -> w660
              tunnel: w659 -> [w666 w668]
              tunnel: w658 -> [w663 _]
              tunnel: [w662 w667] -> w657
              tunnel: w656 -> [_ w667]
              tunnel: w655 -> [w661 _]
              frame False {
                n188 = call "Read_Characters_From_File.ph.vi"("file path (dialog if empty)"=w663, "start of read offset (chars.: 0)"=w661) -> ("character string"=w665:string, "EOF?"=w662:bool)  [unwired: 1 in, 5 out]
                n189 = Concatenate Strings(w666, w665) -> (w664:string)
              }
              frame True {
              }
            }
          }
          frame "Raw Data File" {
          }
        }
        n190 = Spreadsheet String To Array(format string="%s", spreadsheet string=w648, array type (2D Dbl)=string[][] [] ("Channel Values")) -> (array=w649:string[][])  [unwired: 1 out]
      }
      frame "Delete First Row?" {
        n191 = global read "Results_plotter_Global.vi" "Extra Channel Names"() -> (w683:string[])
        n192 = case shown="True" w671 {
          tunnel: w685 -> [_ w696]
          tunnel: w684 -> [w693 w695]
          tunnel: [w693 w694] -> w676
          frame False {
          }
          frame True {
            n193 = call "Delete_First_Rows.vi"("Data In"=w695, "File Type"=w696) -> ("Data Out"=w694:string[][])  [unwired: 1 out]
          }
        }
        n194 = Array Size(array=w683) -> (size(s)=w682:i32)
        n195 = Greater Than 0?(x=w682) -> (x > 0?=w681:bool)
        n196 = And(x=w671, y=w681) -> (x .and. y?=w680:bool)
        n197 = Array Size(array=w676) -> (size(s)=w675:i32[])
        n198 = Index Array(array=w675, index=0) -> (element=w673:i32)
        n199 = for {
          N: w673 -> [_]
          tunnel: [w692] -> w672 mode=indexing
          i -> [w692]
        }
      }
      frame "Add Extra Channels of data" {
        n200 = global read "Results_plotter_Global.vi" "Extra Channel Names"() -> (w706:string[])
        n201 = global read "Results_plotter_Global.vi" "Extra Channel Values"() -> (w704:string[])
        n202 = for {
          tunnel: w706 -> [w724] mode=indexing
          shift-right: [w722] -> w702
          shift-left: string[] [] -> [w723]
          shift-right: [w725] -> w705
          shift-left: w708 -> [w720]
          tunnel: w704 -> [w721] mode=indexing
          n203 = Search 1D Array(1D array=w720, element=w724) -> (index of element=w719:i32)  [unwired: 1 out]
          n204 = case shown="0, Default" w719 {
            tunnel: w720 -> [w730 w736]
            tunnel: [w730 w735] -> w725
            tunnel: w724 -> [_ w734]
            tunnel: w723 -> [w729 w733]
            tunnel: [w728 w732] -> w722
            tunnel: w721 -> [w726 w731]
            tunnel: w719 -> [w727 _]
            frame 0, Default {
              n205 = Replace Array Subset(array=w729, new element=w726, index=w727) -> (w728:string[])
            }
            frame -1 {
              n206 = Build Array (concatenate)(w736, w734) -> (w735:string[])
              n207 = Build Array (concatenate)(w733, w731) -> (w732:string[])
            }
          }
        }
        n208 = for {
          tunnel: w703 -> [w716] mode=indexing
          tunnel: w702 -> [w718]
          tunnel: [w717] -> w701 mode=indexing
          n209 = Build Array (concatenate)(w716, w718) -> (w717:string[])
        }
      }
    }
    "Case" <- w39
  }
  "Filetype" <- w14
  "Results file Out" <- w12
  "Ch names Out" <- w11
  "Channel Values Out" <- w10
  "String Before" <- w9
  "String After" <- w7
  "Template File Out" <- w6
  "EOF?" <- w4
  "mark after read (chars.)" <- w3
  "Row numbers" <- w2
